vi "Split merged cubes.vi"(8 "Cube 2":T2={"X Min"=10, "X Max"=11, "Y Min"=10, "Y Max"=11, "Z Min"=10, "Z Max"=11}, 11 "Cube 1":T2={"X Min"=0, "X Max"=10, "Y Min"=0, "Y Max"=10, "Z Min"=0, "Z Max"=10}) -> (3 "Splitted Cubes":T1(array[cluster]))   [LabVIEW 2021]
uses:
  <vilib>/Comparison/Less/Less Functor/Less Functor.lvclass
panel:
  out "size(s)":i32
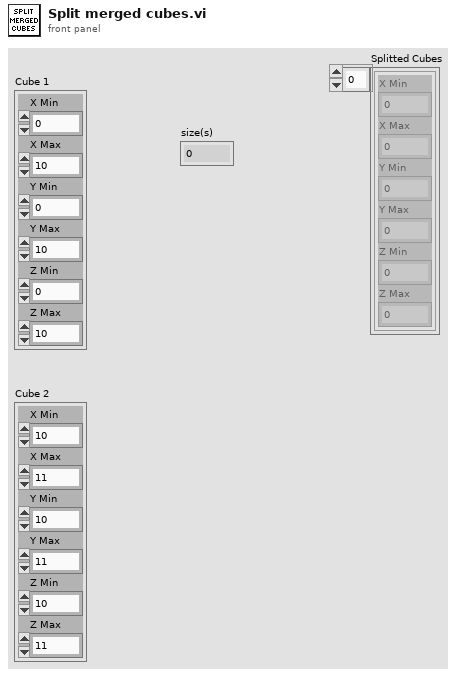
[diagram p1: front panel]
types:
  T1 = cluster{"X Min":i64, "X Max":i64, "Y Min":i64, "Y Max":i64, "Z Min":i64, "Z Max":i64}[]
  T2 = cluster{"X Min":i64, "X Max":i64, "Y Min":i64, "Y Max":i64, "Z Min":i64, "Z Max":i64}
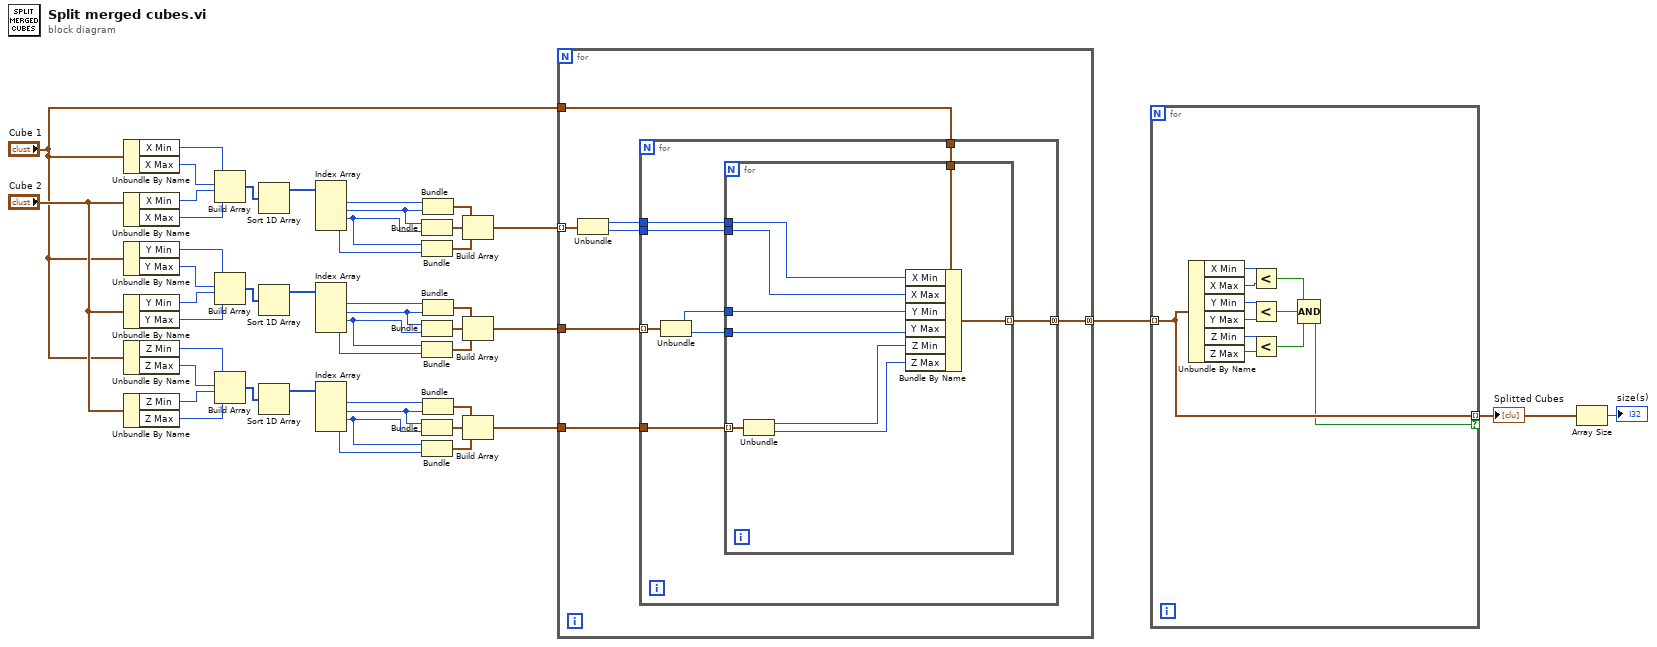
[diagram p0: block diagram]
diagram:
  n1 = Unbundle By Name("Cube 1") -> ("X Min"=w47:i64, "X Max"=w46:i64)
  n2 = Unbundle By Name("Cube 2") -> ("X Min"=w45:i64, "X Max"=w44:i64)
  n3 = Unbundle By Name("Cube 1") -> ("Y Min"=w36:i64, "Y Max"=w37:i64)
  n4 = Unbundle By Name("Cube 2") -> ("Y Min"=w38:i64, "Y Max"=w39:i64)
  n5 = Unbundle By Name("Cube 1") -> ("Z Min"=w35:i64, "Z Max"=w34:i64)
  n6 = Unbundle By Name("Cube 2") -> ("Z Min"=w33:i64, "Z Max"=w32:i64)
  n7 = Build Array(w47, w46, w45, w44) -> (w43:i64[])
  n8 = Build Array(w36, w37, w38, w39) -> (w40:i64[])
  n9 = Build Array(w35, w34, w33, w32) -> (w31:i64[])
  n10 = Sort 1D Array(array=w43) -> (sorted array=w42:i64[])
  n11 = Sort 1D Array(array=w40) -> (sorted array=w41:i64[])
  n12 = Sort 1D Array(array=w31) -> (sorted array=w30:i64[])
  n13 = Index Array(array=w42) -> (element #1=w28:i64, element #2=w9:i64, element #3=w10:i64, element #4=w11:i64)  [unwired: 4 in]
  n14 = Index Array(array=w41) -> (element #1=w21:i64, element #2=w6:i64, element #3=w7:i64, element #4=w8:i64)  [unwired: 4 in]
  n15 = Index Array(array=w30) -> (element #1=w17:i64, element #2=w3:i64, element #3=w4:i64, element #4=w5:i64)  [unwired: 4 in]
  n16 = Bundle("X Max"=w9, "X Max"=w10) -> (w26:cluster{"X Max":i64, "X Max":i64})  [unwired: 1 in]
  n17 = Bundle("X Max"=w10, "X Max"=w11) -> (w27:cluster{"X Max":i64, "X Max":i64})  [unwired: 1 in]
  n18 = Bundle("Y Max"=w6, "Y Max"=w7) -> (w23:cluster{"Y Max":i64, "Y Max":i64})  [unwired: 1 in]
  n19 = Bundle("Y Max"=w7, "Y Max"=w8) -> (w22:cluster{"Y Max":i64, "Y Max":i64})  [unwired: 1 in]
  n20 = Bundle("Z Max"=w3, "Z Max"=w4) -> (w19:cluster{"Z Max":i64, "Z Max":i64})  [unwired: 1 in]
  n21 = Bundle("Z Max"=w4, "Z Max"=w5) -> (w20:cluster{"Z Max":i64, "Z Max":i64})  [unwired: 1 in]
  n22 = Bundle("X Max"=w28, "X Max"=w9) -> (w25:cluster{"X Max":i64, "X Max":i64})  [unwired: 1 in]
  n23 = Bundle("Y Max"=w21, "Y Max"=w6) -> (w24:cluster{"Y Max":i64, "Y Max":i64})  [unwired: 1 in]
  n24 = Bundle("Z Max"=w17, "Z Max"=w3) -> (w18:cluster{"Z Max":i64, "Z Max":i64})  [unwired: 1 in]
  n25 = Build Array(w25, w26, w27) -> (w16:cluster{"X Max":i64, "X Max":i64}[])
  n26 = Build Array(w24, w23, w22) -> (w15:cluster{"Y Max":i64, "Y Max":i64}[])
  n27 = Build Array(w18, w19, w20) -> (w14:cluster{"Z Max":i64, "Z Max":i64}[])
  n28 = for {
    tunnel: w16 -> [w52] mode=indexing
    tunnel: w15 -> [w54]
    tunnel: w14 -> [w53]
    tunnel: "Cube 1" -> [w51]
    tunnel: [w50] -> w2 mode=concatenating
    n29 = Unbundle(w52) -> ("X Max"=w49:i64, "X Max"=w48:i64)
    n30 = for {
      tunnel: w54 -> [w61] mode=indexing
      tunnel: w53 -> [w62]
      tunnel: w51 -> [w60]
      tunnel: w48 -> [w59]
      tunnel: w49 -> [w58]
      tunnel: [w57] -> w50 mode=concatenating
      n31 = Unbundle(w61) -> ("Y Max"=w56:i64, "Y Max"=w55:i64)
      n32 = for {
        tunnel: w62 -> [w71] mode=indexing
        tunnel: w60 -> [w70]
        tunnel: w55 -> [w69]
        tunnel: w56 -> [w68]
        tunnel: w59 -> [w67]
        tunnel: w58 -> [w66]
        tunnel: [w65] -> w57 mode=indexing
        n33 = Unbundle(w71) -> ("Z Max"=w64:i64, "Z Max"=w63:i64)
        n34 = Bundle By Name(cluster=w70, "X Min"=w66, "X Max"=w67, "Y Min"=w68, "Y Max"=w69, "Z Min"=w64, "Z Max"=w63) -> (w65:T2)
      }
    }
  }
  n35 = for {
    tunnel: w2 -> [w73] mode=indexing
    tunnel: [w73] -> w1 mode=indexing if=w72
    n36 = Unbundle By Name(w73) -> ("X Min"=w80:i64, "X Max"=w79:i64, "Y Min"=w78:i64, "Y Max"=w77:i64, "Z Min"=w81:i64, "Z Max"=w82:i64)
    n37 = Less?(x=w80, y=w79) -> (x < y?=w74:bool)
    n38 = Less?(x=w78, y=w77) -> (x < y?=w75:bool)
    n39 = Less?(x=w81, y=w82) -> (x < y?=w76:bool)
    n40 = Compound Arithmetic op=AND(w74, w75, w76) -> (w72:bool)
  }
  "Splitted Cubes" <- w1
  n41 = Array Size(array=w1) -> (size(s)=→"size(s)":i32)
